vi "SeekerSim.vi"() -> ()   [LabVIEW 2017]
panel:
  out "Direction":dbl(knob) scale=-1.0..1.0
  out "Distance":dbl
  in  "Ty":dbl(slide) scale=-21.0..21.0
  in  "Ta":dbl
  in  "Tx":dbl(slide) scale=-27.0..27.0
  in  "Target Area":dbl=0.6
  in  "Translation Deadband":dbl=0.2
  in  "kPAim":dbl=0.045
  in  "kPDrive":dbl=0.09
  in  "Target height":dbl=1.4
  in  "Camera height":dbl=0.3
  in  "Camera angle":dbl=14.5
  in  "AimMin":dbl
  out "PosOutPlus":dbl
  out "PosOutMin":dbl
  out "LeftFOV":bool
  out "NegOutMin":dbl
  out "NegOutPlus":dbl
  out "RightFOV":bool
  out "Deadband":bool
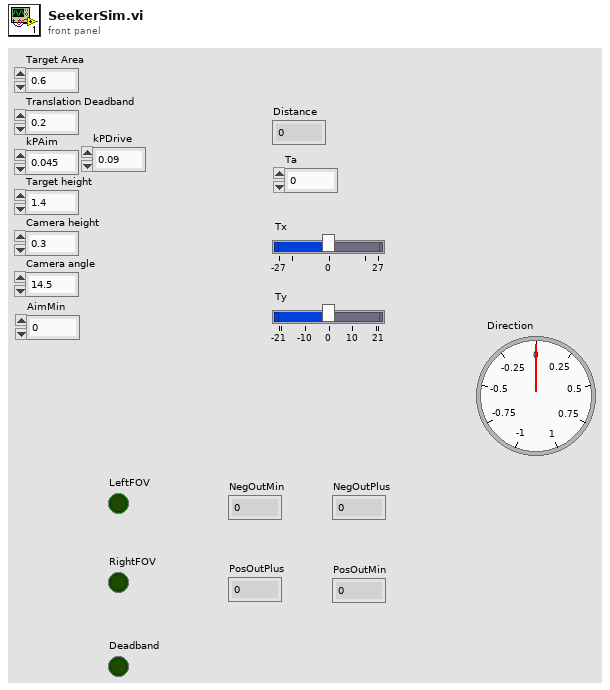
[diagram p1: front panel]
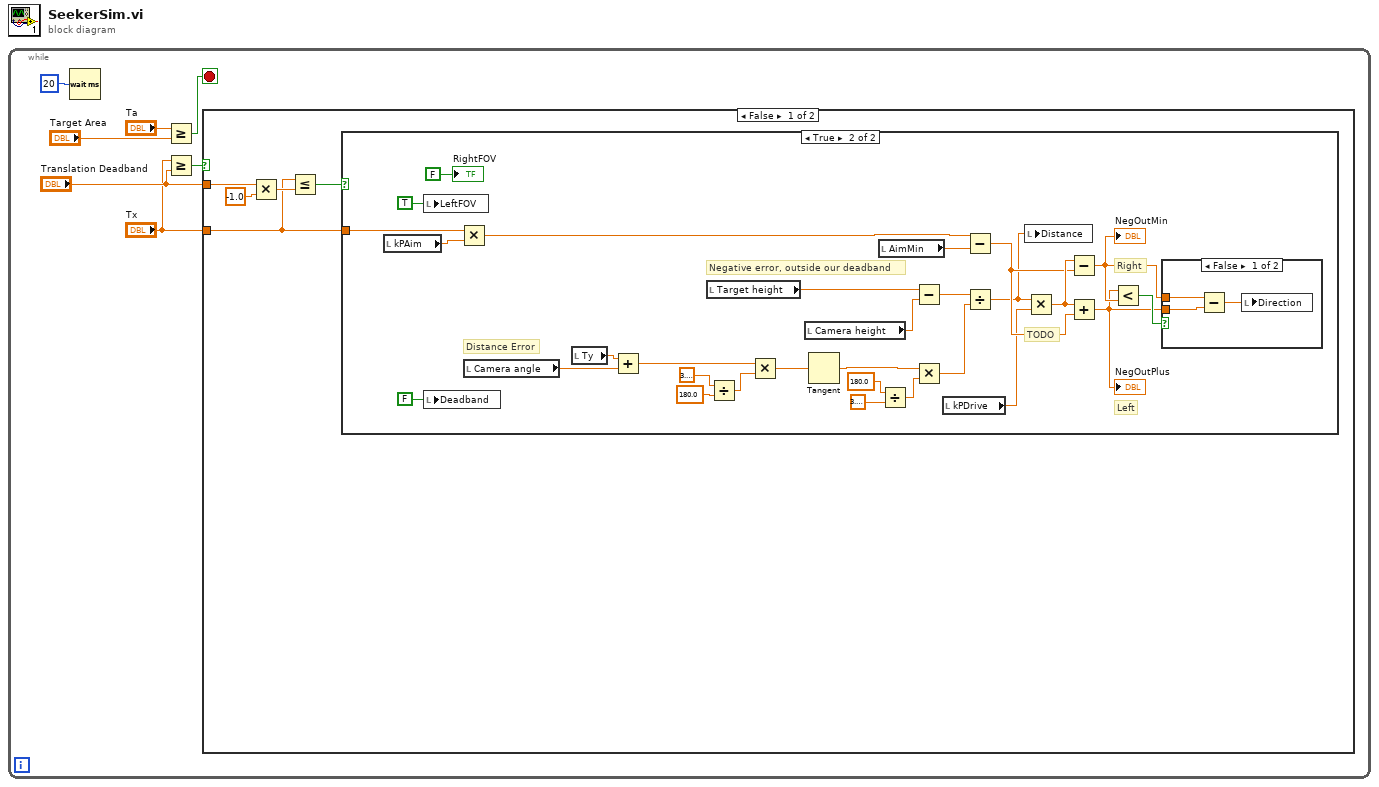
[diagram p0: block diagram]
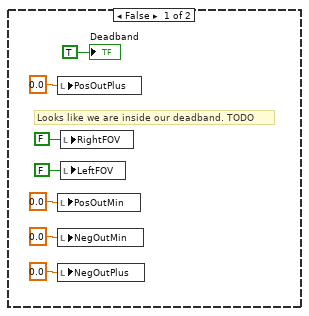
[diagram p2: hidden frame]
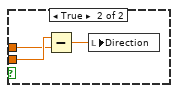
[diagram p3: hidden frame]
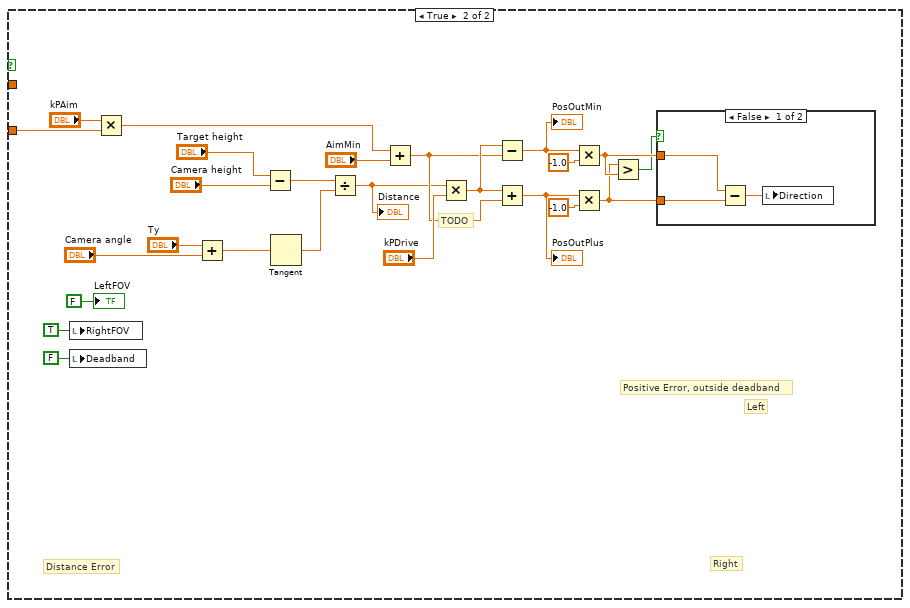
[diagram p4: hidden frame]
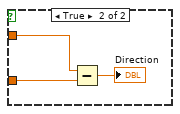
[diagram p5: hidden frame]
diagram:
  n1 = while {
    stop <- w5 stop-if-true
    n2 = Wait (ms)(milliseconds to wait=u32 20) -> ()  [unwired: 1 out]
    n3 = Greater Or Equal?(x="Ta", y="Target Area") -> (x >= y?=w5:bool)
    n4 = Greater Or Equal?(x="Tx", y="Translation Deadband") -> (x >= y?=w4:bool)
    n5 = case shown="False" w4 {
      tunnel: "Tx" -> [w8 w79]
      tunnel: "Translation Deadband" -> [w10 _]
      frame False {
        n6 = Multiply(x=w10, y=-1.0) -> (x*y=w11:dbl)
        n7 = Less Or Equal?(x=w8, y=w11) -> (x <= y?=w9:bool)
        n8 = case shown="True" w9 {
          tunnel: w8 -> [_ w40]
          frame False {
            # "Looks like we are inside our deadband. TODO"
            n9 = local write "PosOutPlus"(0.0 ("NegOutMin")) -> ()
            n10 = local write "PosOutMin"(0.0 ("NegOutMin")) -> ()
            n11 = local write "NegOutMin"(0.0 ("NegOutMin")) -> ()
            n12 = local write "NegOutPlus"(0.0 ("NegOutMin")) -> ()
            n13 = local write "RightFOV"(FALSE ("RightFOV")) -> ()
            n14 = local write "LeftFOV"(FALSE ("LeftFOV")) -> ()
            "Deadband" <- TRUE ("Deadband")
          }
          frame True {
            # "Right"
            # "Left"
            # "TODO"
            # "Distance Error"
            # "Negative error, outside our deadband"
            n15 = local read "kPAim"() -> (w39:dbl)
            n16 = local write "LeftFOV"(TRUE ("LeftFOV")) -> ()
            n17 = local write "Deadband"(FALSE ("Deadband")) -> ()
            n18 = Multiply(x=w40, y=w39) -> (x*y=w47:dbl)
            n19 = local read "Camera angle"() -> (w42:dbl)
            n20 = local read "Ty"() -> (w33:dbl)
            n21 = Add(x=w33, y=w42) -> (x+y=w26:dbl)
            n22 = local read "Target height"() -> (w44:dbl)
            n23 = Divide(x=3.141592653589793, y=180.0) -> (x/y=w27:dbl)
            n24 = Multiply(x=w26, y=w27) -> (x*y=w25:dbl)
            n25 = local read "Camera height"() -> (w43:dbl)
            n26 = Tangent(1:w25) -> (0:w21:dbl)
            n27 = local read "AimMin"() -> (w38:dbl)
            n28 = Divide(x=180.0, y=3.141592653589793) -> (x/y=w22:dbl)
            n29 = Subtract(x=w44, y=w43) -> (x-y=w48:dbl)
            n30 = Multiply(x=w21, y=w22) -> (x*y=w20:dbl)
            n31 = local read "kPDrive"() -> (w41:dbl)
            n32 = Subtract(x=w47, y=w38) -> (x-y=w45:dbl)
            n33 = Divide(x=w48, y=w20) -> (x/y=w34:dbl)
            n34 = local write "Distance"(w34) -> ()
            n35 = Multiply(x=w34, y=w41) -> (x*y=w46:dbl)
            n36 = Subtract(x=w46, y=w45) -> (x-y=w31:dbl)
            "NegOutMin" <- w31
            n37 = Add(x=w46, y=w45) -> (x+y=w30:dbl)
            "NegOutPlus" <- w30
            n38 = Less?(x=w30, y=w31) -> (x < y?=w32:bool)
            n39 = case shown="False" w32 {
              tunnel: w31 -> [w51 w52]
              tunnel: w30 -> [w50 w53]
              frame False {
                n40 = Subtract(x=w51, y=w50) -> (x-y=w49:dbl)
                n41 = local write "Direction"(w49) -> ()
              }
              frame True {
                n42 = Subtract(x=w53, y=w52) -> (x-y=w54:dbl)
                n43 = local write "Direction"(w54) -> ()
              }
            }
            "RightFOV" <- FALSE ("RightFOV")
          }
        }
      }
      frame True {
        # "Left"
        # "Right"
        # "TODO"
        # "Distance Error"
        # "Positive Error, outside deadband"
        n44 = local write "RightFOV"(TRUE ("RightFOV")) -> ()
        n45 = local write "Deadband"(FALSE ("Deadband")) -> ()
        n46 = Multiply(x="kPAim", y=w79) -> (x*y=w70:dbl)
        n47 = Add(x="Ty", y="Camera angle") -> (x+y=w73:dbl)
        n48 = Subtract(x="Target height", y="Camera height") -> (x-y=w72:dbl)
        n49 = Tangent(1:w73) -> (0:w71:dbl)
        n50 = Divide(x=w72, y=w71) -> (x/y=w62:dbl)
        "Distance" <- w62
        n51 = Add(x=w70, y="AimMin") -> (x+y=w67:dbl)
        n52 = Multiply(x=w62, y="kPDrive") -> (x*y=w68:dbl)
        n53 = Subtract(x=w68, y=w67) -> (x-y=w60:dbl)
        "PosOutMin" <- w60
        n54 = Add(x=w68, y=w67) -> (x+y=w58:dbl)
        "PosOutPlus" <- w58
        n55 = Multiply(x=w60, y=-1.0) -> (x*y=w57:dbl)
        n56 = Multiply(x=w58, y=-1.0) -> (x*y=w56:dbl)
        n57 = Greater?(x=w56, y=w57) -> (0:w55:bool)
        n58 = case shown="False" w55 {
          tunnel: w57 -> [w82 w84]
          tunnel: w56 -> [w81 w83]
          frame False {
            n59 = Subtract(x=w82, y=w81) -> (x-y=w80:dbl)
            n60 = local write "Direction"(w80) -> ()
          }
          frame True {
            n61 = Subtract(x=w84, y=w83) -> (x-y=→"Direction":dbl)
          }
        }
        "LeftFOV" <- FALSE ("LeftFOV")
      }
    }
  }
